vi "Lissajous.vi"() -> ()   [LabVIEW 2017]
panel:
  out "XY Graph":cluster{"Y":dbl[], "Y":dbl[]}[](graph)
  in  "N":dbl
  in  "phi_2":dbl
  in  "phi_1":dbl
  in  "f_2":dbl
  in  "f_1":dbl
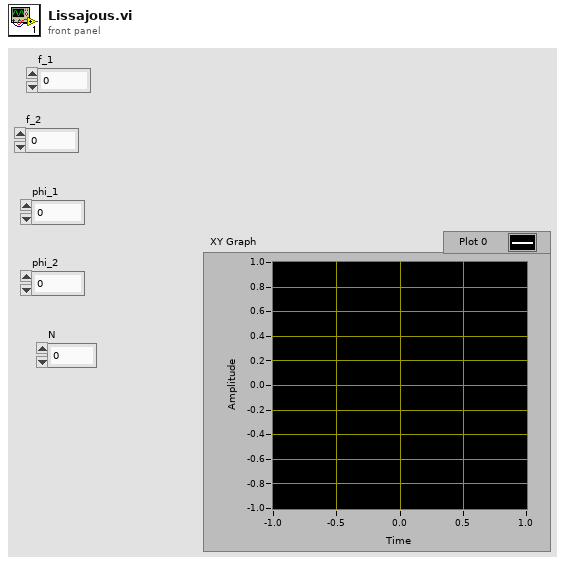
[diagram p1: front panel]
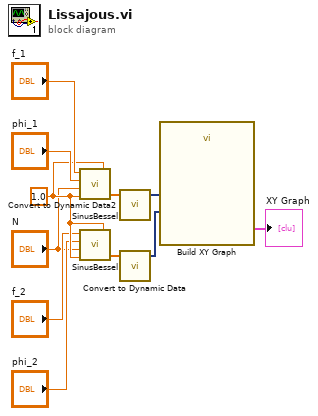
[diagram p0: block diagram]
diagram:
  w4 = 1.0
  n1 = call "SinusBessel.vi"("Amplitude A"=w4, "Bessel v"=w4, "Zahl der Punkte N"="N", "Phase phi"="phi_1", "Frequenz f"="f_1") -> ("y"=w8:dbl[])  [unwired: 1 out]
  n2 = call "SinusBessel.vi"("Amplitude A"=w4, "Bessel v"=w4, "Zahl der Punkte N"="N", "Phase phi"="phi_2", "Frequenz f"="f_2") -> ("y"=w10:dbl[])  [unwired: 1 out]
  n3 = call "Convert to Dynamic Data2"("Array"=w8) -> ("Dynamic Data Type"=w7:dynamicdata)  [unwired: 3 in]
  n4 = call "Convert to Dynamic Data"("Array"=w10) -> ("Dynamic Data Type"=w9:dynamicdata)  [unwired: 3 in]
  n5 = call "Build XY Graph"("Y Input"=w9, "X Input"=w7) -> ("XY Graph"=→"XY Graph":cluster{"X":dbl[], "Y":dbl[]}[])  [unwired: 8 in, 1 out]
